vi "Transfer Function PtByPt.vi"(4 "initialize":bool, 5 "sample length":i32=100, 6 "dt":dbl=1.0 format="%0.2f", 7 "response signal y":dbl format="%0.2f", 8 "stimulus signal x":dbl format="%0.2f") -> (0 "error":i32, 1 "df":dbl format="%0.2f", 2 "Frequency Response Phase (radians)":dbl[](array[numeric]), 3 "Frequency Response Mag (gain)":dbl[](array[numeric]))   [LabVIEW 2020, in "NI_PtbyPt.lvlib"]
doc: "Computes the single-sided transfer function, also known as the frequency response, from the time-domain Stimulus Signal and Response Signal from a network under test."
uses:
  <vilib>/ptbypt/NI_PtbyPt.lvlib
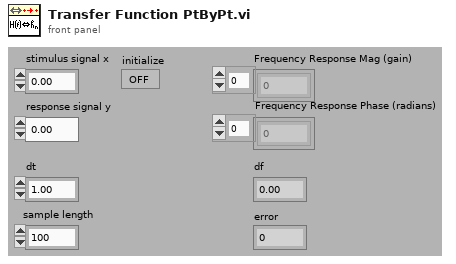
[diagram p1: front panel]
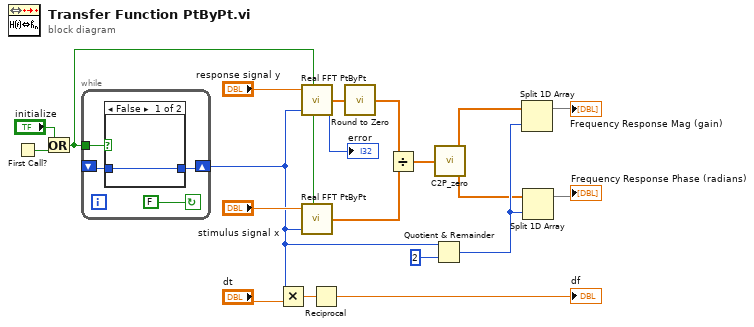
[diagram p0: block diagram]
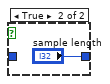
[diagram p2: hidden frame]
diagram:
  n1 = First Call?() -> (First Call?: T/F=w4:bool)
  n2 = Or(x="initialize", y=w4) -> (x .or. y?=w2:bool)
  n3 = while {
    tunnel: w2 -> [w22]
    shift-left: _ -> [w23]
    shift-right: [w24] -> w1
    stop <- FALSE continue-if-true
    n4 = case shown="False" w22 {
      tunnel: [w25 "sample length"] -> w24
      tunnel: w23 -> [w25 _]
      frame False {
      }
      frame True {
      }
    }
  }
  n5 = Multiply(x=w1, y="dt") -> (x*y=w20:dbl)
  n6 = call <vilib>:"Real FFT PtByPt.vi"("initialize"=w2, "sample length"=w1, "x"="response signal y") -> ("error"=→"error":i32, "FFT{X}"=w8:cdb[])  [unwired: 1 in]
  n7 = call <vilib>:"Real FFT PtByPt.vi"("initialize"=w2, "sample length"=w1, "x"="stimulus signal x") -> ("FFT{X}"=w11:cdb[])  [unwired: 1 in, 1 out]
  n8 = Reciprocal(x=w20) -> (1/x=→"df":dbl)
  n9 = call <vilib>:"Round to Zero.vi"("complex"=w8) -> ("result"=w7:cdb[])
  n10 = Divide(x=w7, y=w11) -> (x/y=w9:cdb[])
  n11 = Quotient & Remainder(x=w1, y=2) -> (floor(x/y)=w12:i32)  [unwired: 1 out]
  n12 = call <vilib>:"C2P_zero.vi"("r * e^(i*theta)"=w9) -> ("amplitude"=w6:dbl[], "phase"=w5:dbl[])
  n13 = Split 1D Array(array=w6, index=w12) -> (first subarray=→"Frequency Response Mag (gain)":dbl[])  [unwired: 1 out]
  n14 = Split 1D Array(array=w5, index=w12) -> (first subarray=→"Frequency Response Phase (radians)":dbl[])  [unwired: 1 out]
